vi "relay_action.vi"(0 "relay session in":T1={"VISA resource out"="COM12", "error out"={"status"=FALSE, "code"=0, "source"=""}}, 3 "Action":u8(ring) items=["open dump on"=8, "pump acid on"=9, "air flush on"=10, "stop gas flow on"=11, "open dump off"=0, "pump acid off"=1, "air flush off"=2, "stop gas flow off"=3, "OpenAll"=30, "CloseAll"=29]) -> (6 "relay session out":T1={"VISA resource out"="COM12", "error out"={"status"=FALSE, "code"=0, "source"=""}})   [LabVIEW 2010]
panel:
  out "code":u8=254
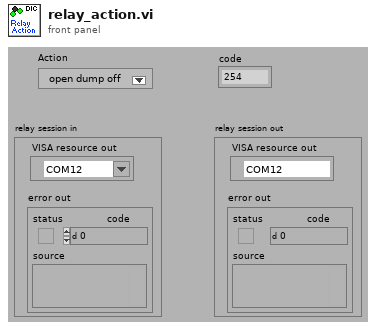
[diagram p1: front panel]
types:
  T1 = cluster{"VISA resource out":refnum<visa-resource-name>, "error out":errorcluster}
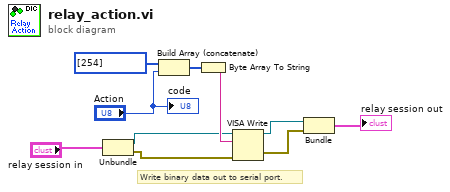
[diagram p0: block diagram]
diagram:
  # "Write binary data out to serial port."
  n1 = Unbundle("relay session in") -> ("VISA resource out"=w5:refnum<visa-resource-name>, "error out"=w4:errorcluster)
  n2 = Build Array (concatenate)(u8[] [254] ("unsigned byte array"), "Action") -> (w8:u8[])
  n3 = Byte Array To String(unsigned byte array=w8) -> (string=w10:string)
  n4 = VISA Write(VISA resource name=w5, write buffer=w10, error in (no error)=w4) -> (VISA resource name out=w2:refnum<visa-resource-name>, error out=w1:errorcluster)  [unwired: 1 out]
  n5 = Bundle("VISA resource out"=w2, "error out"=w1) -> (→"relay session out":T1)  [unwired: 1 in]
  "code" <- "Action"
